vi "measure inputs.vi"(8 "error in (no error)":errorcluster, 10 "Sample averaging (1-10)":i32, 11 "App Data":T2) -> (0 "error out":errorcluster, 3 "Analog inputs":T1)   [LabVIEW 2014]
uses:
  Controls/App Data.ctl
  <vilib>/DAQmx/read.llb/DAQmx Read (Analog 1D DBL NChan 1Samp).vi
  <vilib>/DAQmx/read.llb/DAQmx Read (Analog 2D DBL NChan NSamp).vi
  <vilib>/DAQmx/miscellaneous.llb/DAQmx Fill In Error Info.vi
  <resource>/objmgr/daqmx.rc
panel:
  in  "reset x":bool
  out "current position (test)":dbl
  in  "Simulate inputs":T1={"RF out voltage"=0.0, "position voltage"=0.7, "Start switch voltage"=0.0, "Stop switch voltage"=0.0} {"RF out voltage" min=0.0 max=1.0 step=0.05 format="%.2g"; "position voltage" min=0.7 max=6.0 step=0.001 format="%.3g"}
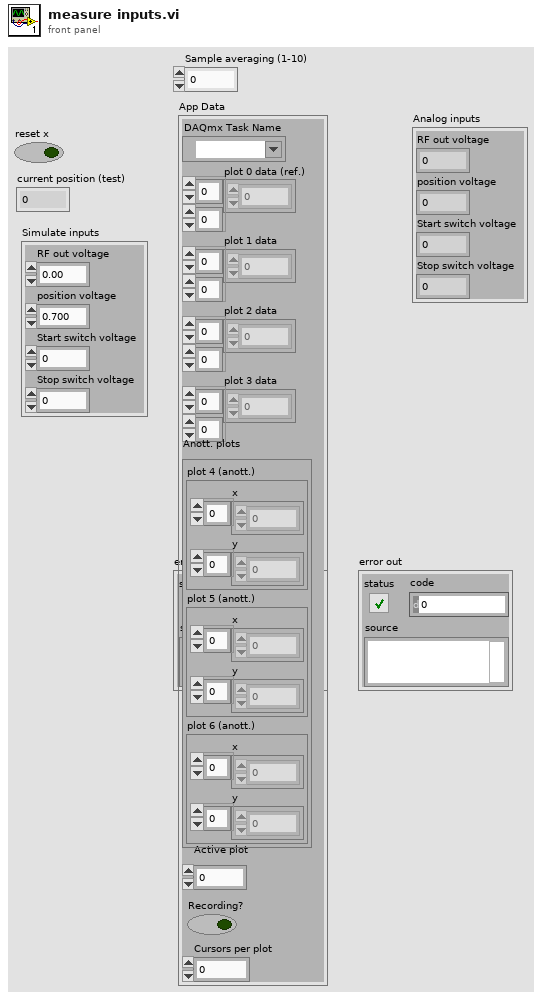
[diagram p1: front panel]
types:
  T1 = cluster{"RF out voltage":dbl, "position voltage":dbl, "Start switch voltage":dbl, "Stop switch voltage":dbl}
  T2 = typedef "App Data.ctl" = cluster{"DAQmx Task Name":refnum<k21>, "plot 0 data (ref.)":dbl[][], "plot 1 data":dbl[][], "plot 2 data":dbl[][], "plot 3 data":dbl[][], "Anott. plots":cluster{"plot 4 (anott.)":cluster{"x":dbl[], "y":dbl[]}, "plot 5 (anott.)":cluster{"x":dbl[], "y":dbl[]}, "plot 6 (anott.)":cluster{"x":dbl[], "y":dbl[]}}, "Active plot":u32, "Recording?":bool, "Cursors per plot":i32}
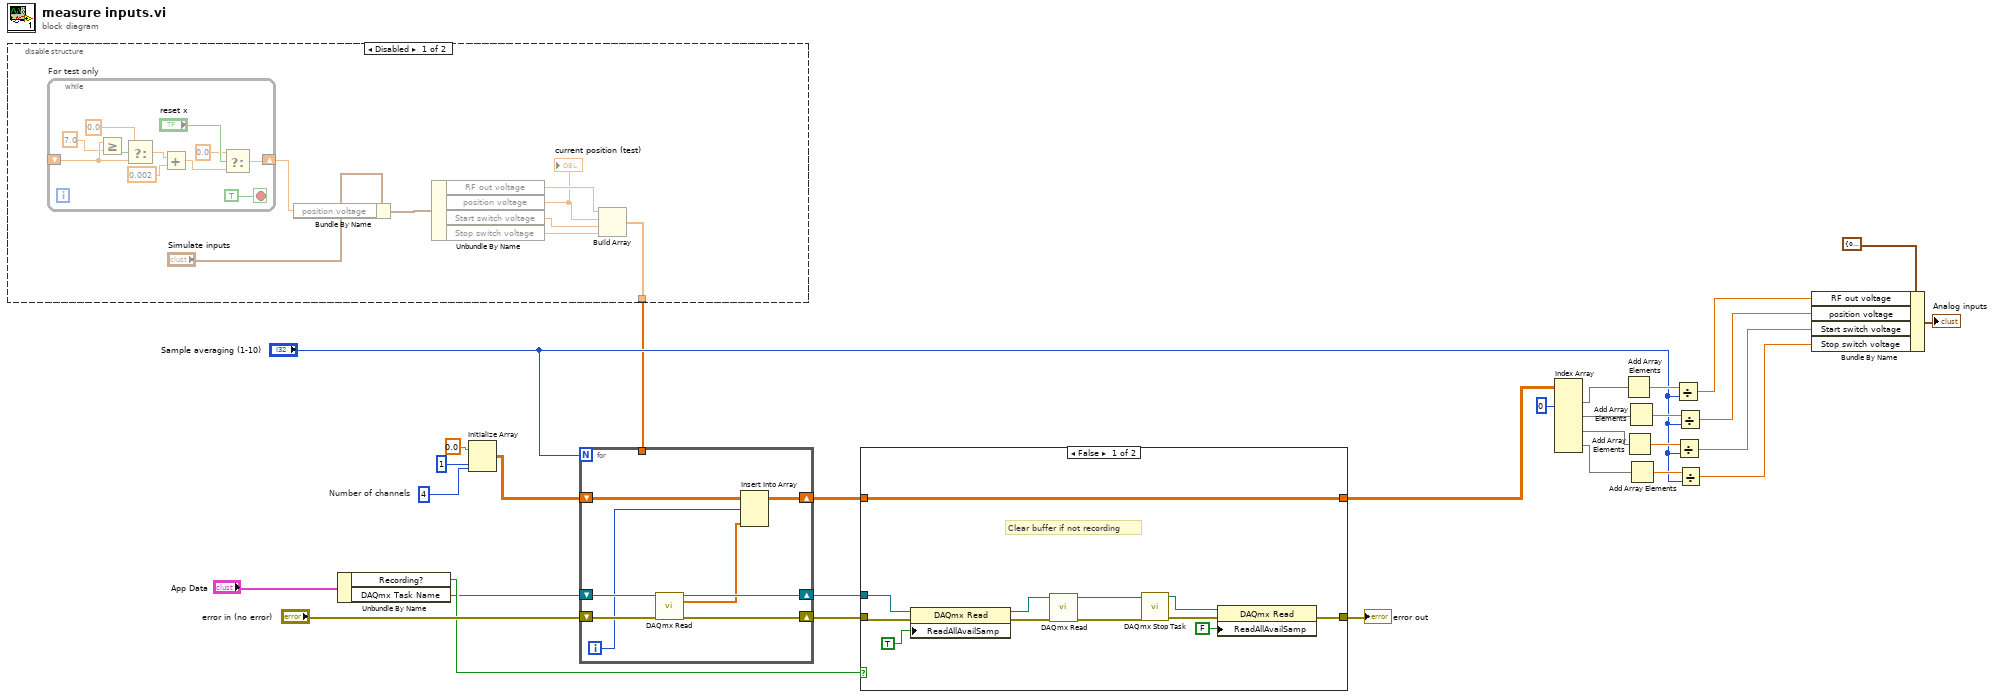
[diagram p0: block diagram]
diagram:
  w11 = 4  # Number of channels
  n1 = disable-structure shown="Disabled" {
    disable-tunnel: [w38 _] -> w4
    frame Disabled {
      n2 = while "For test only" {
        shift-right: [w42] -> w33
        shift-left: _ -> [w44]
        stop <- TRUE stop-if-true
        n3 = Greater Or Equal?(x=w44, y=7.0 ("x")) -> (x >= y?=w47:bool)
        n4 = Select(t=0.0, s=w47, f=w44) -> (s? t:f=w45:dbl)
        n5 = Add(x=w45, y=0.002) -> (x+y=w41:dbl)
        n6 = Select(t=0.0, s="reset x", f=w41) -> (s? t:f=w42:dbl)
      }
      n7 = Bundle By Name(cluster="Simulate inputs", "position voltage"=w33) -> (w31:T1)
      n8 = Unbundle By Name(w31) -> ("RF out voltage"=w37:dbl, "position voltage"=w36:dbl, "Start switch voltage"=w35:dbl, "Stop switch voltage"=w34:dbl)
      "current position (test)" <- w36
      n9 = Build Array(w37, w36, w35, w34) -> (w38:dbl[])
    }
    frame Enabled {
    }
  }
  n10 = Unbundle By Name("App Data") -> ("Recording?"=w8:bool, "DAQmx Task Name"=w1:refnum<k21>)
  n11 = Initialize Array(0.0 ("element"), 1 ("dimension size"), w11) -> (w13:dbl[][])
  n12 = for {
    N: "Sample averaging (1-10)" -> [_]
    shift-right: [w55] -> w7
    shift-left: "error in (no error)" -> [w57]
    shift-right: [w51] -> w5
    shift-left: w1 -> [w56]
    shift-right: [w53] -> w2
    shift-left: w13 -> [w54]
    tunnel: w4 -> [_]
    i -> [w52]
    n13 = call-poly <vilib>:"DAQmx Read.vi"("task/channels in"=w56, "error in"=w57) -> ("task out"=w51:refnum<k21>, "data"=w50:dbl[], "error out"=w55:errorcluster)  [unwired: 11 in]
    n14 = Insert Into Array(array=w54, index (row)=w52, new element=w50) -> (w53:dbl[][])  [unwired: 1 in]
  }
  n15 = case shown="False" w8 {
    tunnel: w7 -> [w61 w71]
    tunnel: [w63 w71] -> w6
    tunnel: w5 -> [w66 _]
    tunnel: [w69 w70] -> w3
    tunnel: w2 -> [w69 w70]
    frame False {
      # "Clear buffer if not recording"
      n16 = property class="DAQmx Read"(reference=w66, error in=w61, "ReadAllAvailSamp"=TRUE) -> (reference out=w65:refnum<k21>, error out=w62:errorcluster)
      n17 = call-poly <vilib>:"DAQmx Read.vi"("task/channels in"=w65, "error in"=w62) -> ("task out"=w64:refnum<k21>, "error out"=w68:errorcluster)  [unwired: 11 in, 1 out]
      n18 = call <vilib>:"DAQmx Stop Task.vi"("task/channels in"=w64, "error in"=w68) -> ("task out"=w58:refnum<k21>, "error out"=w59:errorcluster)  [unwired: 12 in]
      n19 = property class="DAQmx Read"(reference=w58, error in=w59, "ReadAllAvailSamp"=FALSE) -> (error out=w63:errorcluster)  [unwired: 1 out]
    }
    frame True {
    }
  }
  "error out" <- w6
  n20 = Index Array(array=w3, index (col) #1=0 ("disabled index (col)")) -> (element #1=w27:dbl[], element #2=w28:dbl[], element #3=w21:dbl[], element #4=w20:dbl[])  [unwired: 7 in]
  n21 = Add Array Elements(numeric array=w27) -> (sum=w29:dbl)
  n22 = Add Array Elements(numeric array=w21) -> (sum=w23:dbl)
  n23 = Add Array Elements(numeric array=w28) -> (sum=w30:dbl)
  n24 = Add Array Elements(numeric array=w20) -> (sum=w22:dbl)
  n25 = Divide(x=w29, y="Sample averaging (1-10)") -> (x/y=w19:dbl)
  n26 = Divide(x=w23, y="Sample averaging (1-10)") -> (x/y=w17:dbl)
  n27 = Divide(x=w30, y="Sample averaging (1-10)") -> (x/y=w18:dbl)
  n28 = Divide(x=w22, y="Sample averaging (1-10)") -> (x/y=w16:dbl)
  n29 = Bundle By Name(cluster=T1 {"RF out voltage"=0.0, "position voltage"=0.0, "Start switch voltage"=0.0, "Stop switch voltage"=0.0}, "RF out voltage"=w19, "position voltage"=w18, "Start switch voltage"=w17, "Stop switch voltage"=w16) -> (→"Analog inputs":T1)
